vi "_Accept AutoDV results.vi"(8 "error in (no error)":errorcluster, 9 "Run Bias Info":T1[](array[typedef]), 10 "Optimization Run Bias":u32) -> (0 "error out":errorcluster)   [LabVIEW 2015]
uses:
  Controls/Auto-Detector Peak Info.ctl
  <vilib>/Utility/config.llb/Read Key (Path).vi
  <vilib>/Utility/file.llb/Write Delimited Spreadsheet (string).vi
  <vilib>/Utility/config.llb/NI_LVConfig.lvlib
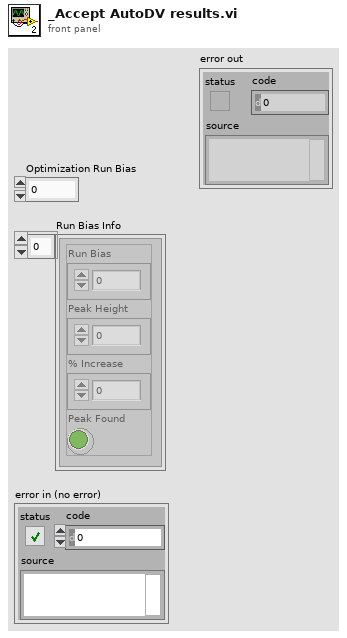
[diagram p1: front panel]
types:
  T1 = typedef "Auto-Detector Peak Info.ctl" = cluster{"Run Bias":u32, "Peak Height":dbl, "% Increase":dbl, "Peak Found":bool}
  T2 = typedef "NI_LVConfig.lvlib/Config Data RefNum.ctl" = refnum<k1>
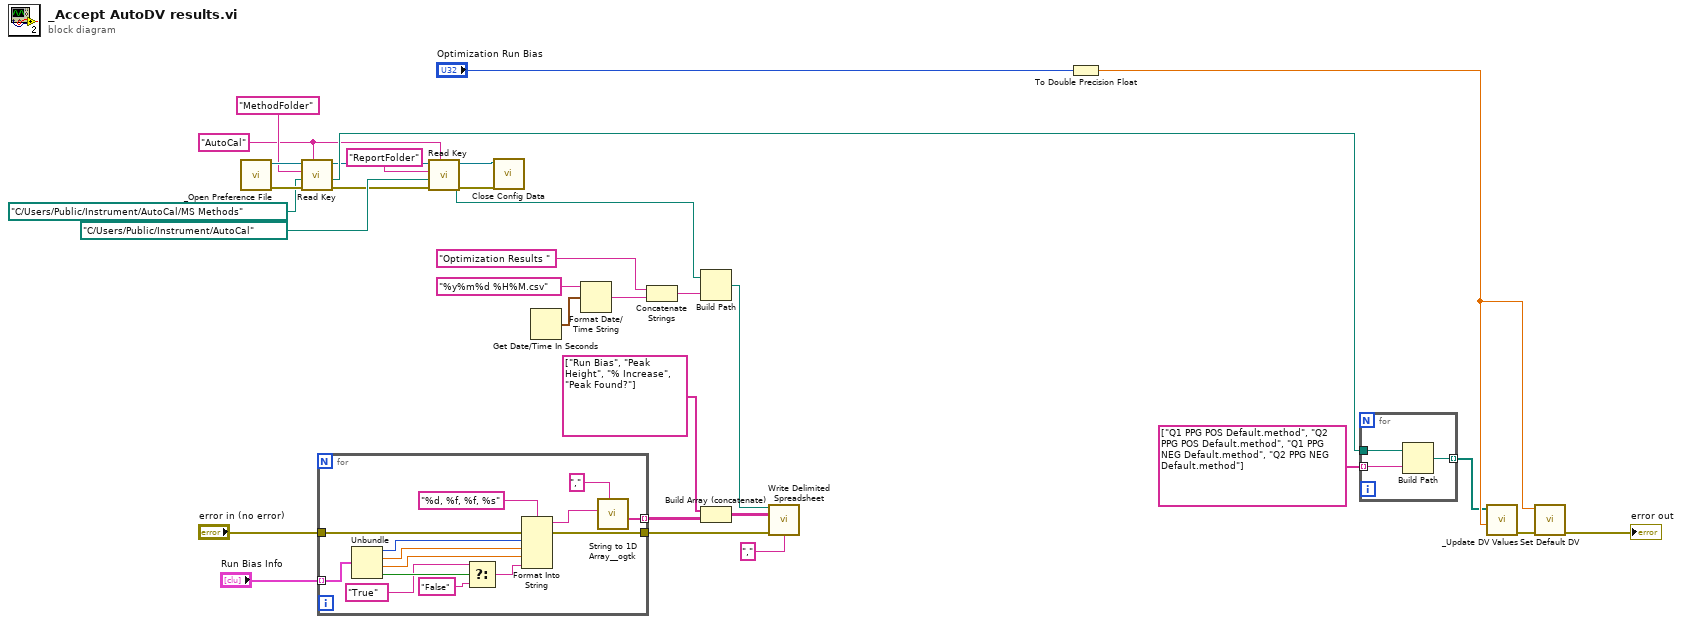
[diagram p0: block diagram]
diagram:
  w7 = "AutoCal" ("section")
  n1 = call "_Open Preference File.vi"() -> ("error"=w14:errorcluster, "refnum"=w16:T2)  [unwired: 3 in, 3 out]
  n2 = call-poly <vilib>:"Read Key.vi"("section"=w7, "error in (no error)"=w14, "default value"=path "C:/Users/Public/Instrument/AutoCal/MS Methods" ("oldTablePath"), "key"="MethodFolder" ("section"), "refnum"=w16) -> ("error out"=w9:errorcluster, "value"=w12:path, "refnum out"=w6:T2)  [unwired: 3 in, 1 out]
  n3 = for {
    tunnel: "Run Bias Info" -> [w46] mode=indexing
    tunnel: "error in (no error)" -> [w37]
    tunnel: [w36] -> w24
    tunnel: [w33] -> w26 mode=indexing
    n4 = Unbundle(w46) -> ("Run Bias"=w45:u32, "Peak Height"=w44:dbl, "% Increase"=w43:dbl, "Peak Found"=w41:bool)
    n5 = Select(t="True", s=w41, f="False") -> (s? t:f=w38:string)
    n6 = Format Into String(format string="%d, %f, %f, %s", error in=w37, w45, w44, w43, w38) -> (resulting string=w35:string, error out=w36:errorcluster)  [unwired: 1 in]
    n7 = call <userlib>:"String to 1D Array__ogtk.vi"("delimiter (Tab)"=",", "string"=w35) -> ("Array of Strings"=w33:string[])  [unwired: 9 in]
  }
  n8 = call-poly <vilib>:"Read Key.vi"("section"=w7, "error in (no error)"=w9, "default value"=path "C:/Users/Public/Instrument/AutoCal" ("path"), "key"="ReportFolder" ("section"), "refnum"=w6) -> ("error out"=w4:errorcluster, "value"=w8:path, "refnum out"=w5:T2)  [unwired: 3 in, 1 out]
  n9 = call <vilib>:"Close Config Data.vi"("error in (no error)"=w4, "refnum"=w5) -> ()  [unwired: 8 in, 2 out]
  n10 = Get Date/Time In Seconds() -> (seconds since 1Jan1904=w30:timestamp)
  n11 = Format Date/Time String(time format string (%c)="%y%m%d %H%M.csv", seconds (now)=w30) -> (date/time string=w32:string)  [unwired: 1 in]
  n12 = Concatenate Strings("Optimization Results " ("name or relative path"), w32) -> (w31:string)
  n13 = Build Path(base path=w8, name or relative path=w31) -> (appended path=w23:path)
  n14 = Build Array (concatenate)(string[] ["Run Bias", "Peak Height", "% Increase", "Peak Found?"], w26) -> (w28:string[][])
  n15 = call-poly <vilib>:"Write Delimited Spreadsheet.vi"("file path (dialog if empty)"=w23, "2D data"=w28, "error in (no error)"=w24, "delimiter (\\t)"="," ("delimiter (\\t)")) -> ()  [unwired: 10 in, 2 out]
  n16 = To Double Precision Float(number="Optimization Run Bias") -> (double precision float=w20:dbl)
  n17 = for {
    tunnel: string[] ["Q1 PPG POS Default.method", "Q2 PPG POS Default.method", "Q1 PPG NEG Default.method", "Q2 PPG NEG Default.method"] -> [w49] mode=indexing
    tunnel: w12 -> [w48]
    tunnel: [w47] -> w3 mode=indexing
    n18 = Build Path(base path=w48, name or relative path=w49) -> (appended path=w47:path)
  }
  n19 = call "_Update DV Values.vi"("UserInput"=w20, "FileNames"=w3) -> ("error out"=w1:errorcluster)  [unwired: 9 in]
  n20 = call "Set Default DV.vi"("error in (no error)"=w1, "DV Default Value"=w20) -> ("error out"=→"error out":errorcluster)  [unwired: 9 in]
